vi "ActionVIOnLoad.vi"(8 "error in (no error)":errorcluster, 11 "Device Item Ref in":T1 format="%.0x") -> (0 "error out":errorcluster, 3 "Device Item Ref out":T1 format="%.0x")   [LabVIEW 2019, in "Profile Interpolation System Explorer.lvlib"]
uses:
  Profile Interpolation System Explorer.lvlib
  <vilib>/NI VeriStand/Custom Device API/Custom Device Item Ref.ctl
  Shared/Types/FG Action.ctl
  Shared/SubVIs/Constants.vi
  <vilib>/NI VeriStand/Custom Device API/NI VeriStand - Get Item Property.vi
  <vilib>/NI VeriStand/Custom Device API/Get Item Property (Path).vi
  <vilib>/NI VeriStand/Custom Device API/Get Item Property (Boolean).vi
  <vilib>/NI VeriStand/Custom Device API/NI VeriStand - Set Item Property.vi
  <vilib>/NI VeriStand/Custom Device API/Set Item Property (Path).vi
  <vilib>/NI VeriStand/Custom Device API/Set Item Property (Boolean).vi
  <vilib>/NI VeriStand/Custom Device Tools/Custom Device Utility Library/NI VeriStand - Search for Item by GUID.vi
  Shared/Profile Interpolation Shared.lvlib
  <vilib>/NI VeriStand/Custom Device API/Custom Device API.lvlib
  <vilib>/NI VeriStand/Custom Device Tools/Custom Device Utility Library/Custom Device Utility Library.lvlib
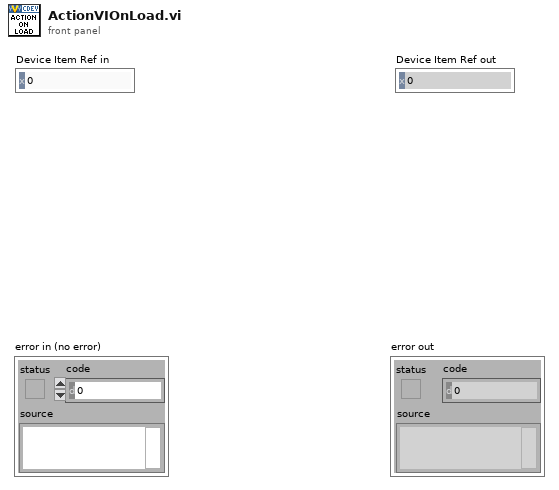
[diagram p1: front panel]
types:
  T1 = typedef "Custom Device API.lvlib/Custom Device Item Ref.ctl" = u64
  T2 = typedef "Profile Interpolation Shared.lvlib/FG Action.ctl" = enum8{"GET", "SET"}
  T3 = typedef "Profile Interpolation Shared.lvlib/Interpolation Settings.ctl" = cluster{"Interpolation File":path, "Create Limit Channels?":bool}
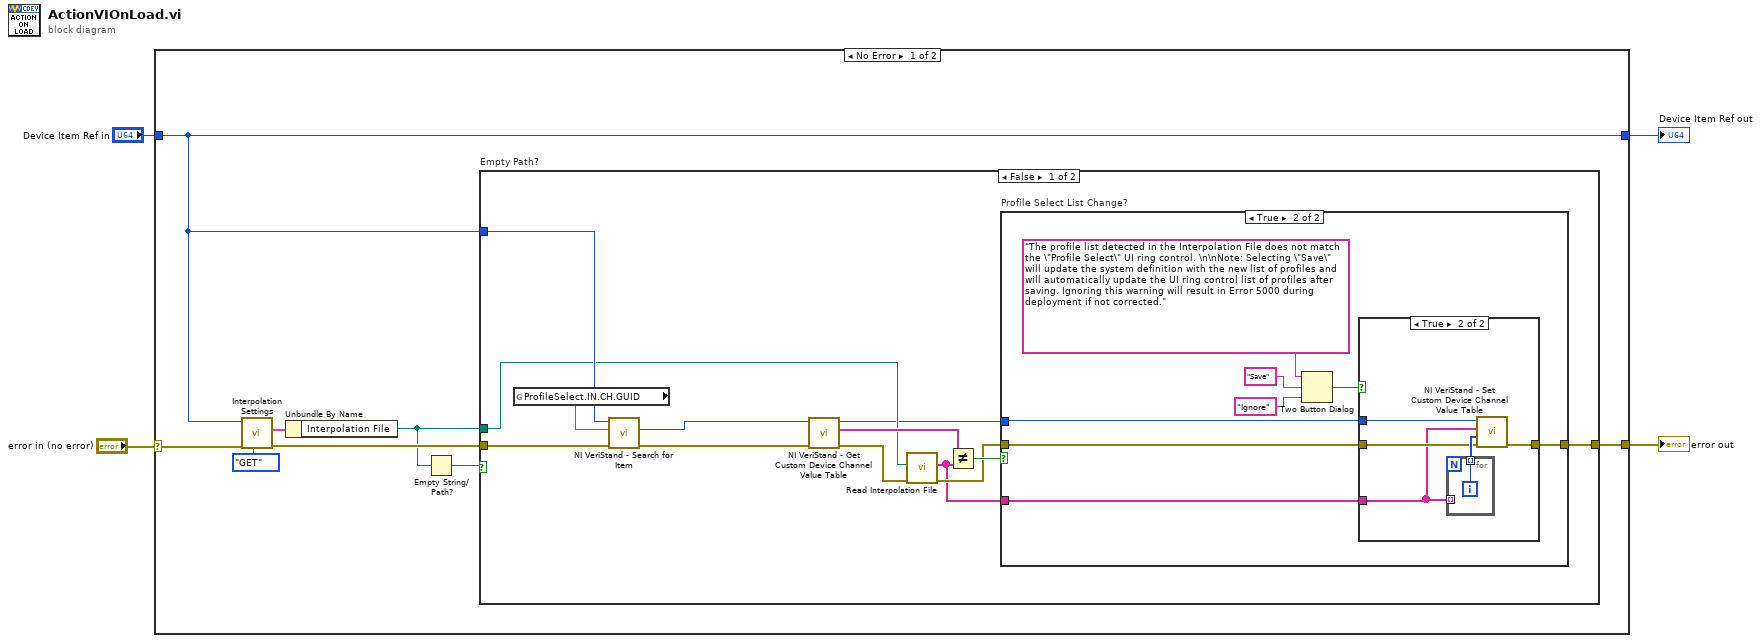
[diagram p0: block diagram]
diagram:
  n1 = case shown="No Error" "error in (no error)" {
    selector: "error in (no error)" -> [w6 w44]
    tunnel: [w10 w44] -> w3
    tunnel: "Device Item Ref in" -> [w5 w43]
    tunnel: [w5 w43] -> w1
    frame No Error {
      n2 = call "Interpolation Settings.vi"("Action"=FG_Action."GET", "error in (no error)"=w6, "Item Ref"=w5) -> ("error out"=w11:errorcluster, "Interpolation Settings out"=w7:T3)  [unwired: 6 in, 1 out]
      n3 = Unbundle By Name(w7) -> ("Interpolation File"=w9:path)
      n4 = Empty String/Path?(string/path=w9) -> (empty?=w8:bool)
      n5 = case "Empty Path?" shown="False" w8 {
        tunnel: w11 -> [w21 w42]
        tunnel: [w23 w42] -> w10
        tunnel: w9 -> [w17 _]
        tunnel: w5 -> [w18 _]
        frame False {
          n6 = global read "Constants.vi" "ProfileSelect.IN.CH.GUID"() -> (w22:string)
          n7 = call-poly <vilib>:"NI VeriStand - Search for Item.vi"("error in"=w21, "Item GUID"=w22, "Section Ref in"=w18) -> ("error out"=w13:errorcluster, "Item Ref"=w14:T1)  [unwired: 5 in, 2 out]
          n8 = call <vilib>:"NI VeriStand - Get Custom Device Channel Value Table.vi"("error in (no error)"=w13, "Channel Ref in"=w14) -> ("error out"=w20:errorcluster, "Names"=w19:string[], "Channel Ref out"=w16:T1)  [unwired: 6 in, 1 out]
          n9 = call "Read Interpolation File.vi"("error in"=w20, "file path (dialog if empty)"=w17) -> ("error out"=w24:errorcluster, "Profiles"=w15:string[])  [unwired: 2 in, 6 out]
          n10 = Not Equal?(x=w19, y=w15) -> (x != y?=w25:bool)
          n11 = case "Profile Select List Change?" shown="True" w25 {
            tunnel: w24 -> [w26 w30]
            tunnel: [w26 w29] -> w23
            tunnel: w16 -> [_ w28]
            tunnel: w15 -> [_ w27]
            frame False {
            }
            frame True {
              n12 = Two Button Dialog(message="The profile list detected in the Interpolation File does not match the \"Profile Select\" UI ring control. \n\nNote: Selecting \"Save\" will update the system definition with the new list of profiles and will automatically update the UI ring control list of profiles after saving. Ignoring this warning will result in Error 5000 during deployment if not corrected.", 1:"Ignore" ("T button name (\"OK\")"), 2:"Save" ("T button name (\"OK\")")) -> (T button?=w31:bool)
              n13 = case shown="True" w31 {
                tunnel: w30 -> [w35 w38]
                tunnel: [w35 w37] -> w29
                tunnel: w28 -> [_ w39]
                tunnel: w27 -> [_ w36]
                frame False {
                }
                frame True {
                  n14 = for {
                    tunnel: [w41] -> w40 mode=indexing
                    tunnel: w36 -> [_] mode=indexing
                    i -> [w41]
                  }
                  n15 = call <vilib>:"NI VeriStand - Set Custom Device Channel Value Table.vi"("error in (no error)"=w38, "Values"=w40, "Names"=w36, "Channel Ref in"=w39) -> ("error out"=w37:errorcluster)  [unwired: 6 in, 1 out]
                }
              }
            }
          }
        }
        frame True {
        }
      }
    }
    frame Error {
    }
  }
  "error out" <- w3
  "Device Item Ref out" <- w1
